vi "GenerateDigitalWaveform.vi"(8 "error in (no error)":errorcluster, 11 "SetupInfo_IN":T1={"ConfigParameters_Analog"={"JAI camera fps"=240.0, "Bi-Lateral Galvo xy scan range (V)"=0.7, "Bi-Lateral Galvo xy scan frequency (Hz)"=500, "AOM Blind percent (%)"=0.1, "AOM start blind percent (%) "=70.0, "ROI threshold"=1.0, "AO Sampling rate"=1000000.0}, "ConfigParameters_Digital"={"Steps per volume"=25.0, "Time per volume (s)"=0.4, "OG start layer"=15.0, "Objective Lin Rising Vel (micron/ms）"=1.0, "Image depth (micron)"=200.0, "OG latency (s)"=10.0, "OG repitation"=3.0, "OG end layer"=17.0, "Shock1 duration (s)"=0.001, "Shock2 duration (s)"=0.001, "Shock3 duration (s)"=0.01, "Shock4 duration (s)"=0.01, "Shock5 duration (s)"=0.1, "Shock duration_New"=[]}, "ConfigParameters_Other1"={"Frontal Galvo xy scan range (V)"=0.14, "Frontal Galvo xy scan frequency (Hz)"=500, "PFI 0 digital clock frequency"=500000.0, "Window size for layer index"=0.5, "sCMOS fps"=95.0}, "ConfigParameters_Others2"={"#Trials baseline"=6, "#Trials test"=6, "Time before acq. (s)"=360.0, "Time before test (s)"=600.0, "#Blocks acquisition"=5, "Inter-trial interval baseline (s)"=60.0, "#Trials per acquition block"=6, "Inter-block interval acquisition (s)"=360.0, "Inter-trial interval acquisition (s)"=20.0, "Flash latency (s)"=10.0, "Flash duration (s)"=3.2, "Response duration (s)"=10.0, "MaxTimeEventDetection (s)"=6, "StimType"=enum."Flash", "#MaxEvents"=6}, "ProcessParametersOut"={"stand Z vol Acquisition time (s)"=0.2631578947368421, "stand Z vol Backward time (s)"=0.13684210526315793, "Objective scan volt"=5.0, "Bi-lateral Galvo Z scan volt"=0.1800000180000018, "Frontal Galvo Z scan volt"=0.14940000509752818, "Objective step length (micron)"=8.0, "OG Z volet Linear Dec time (s)"=0.024, "OG Z vol Stim. steps time (s)"=0.031578947368421054, "OG Z vol Linear Acc time (s)"=0.112, "#Vol. of flash"=8, "#Vol. of shock"=1, "#Vol. bef flash"=25, "#Vol. aft flash"=17, "OG Z vol Linear Dec time (s)"=0.112, "OG Z vol time (s)"=0.39073684210526316, "Stack duration"=[0.001, 0.001, 0.01, 0.01, 0.1], "AOM stand. value size"=400000, "Plane indexing length"=0, "#Vol. blank"=0, "#Vol. blank before acq"=0, "#Vol. blank before test"=0, " #Inter-block interval acquisition (Ed-St Vol)"=0}, "WaveformParameters"={"stand Z vol Acquisition samp info"={"Fs"=1000000.0, "#s"=263158.0}, "stand Z vol Backward samp info"={"Fs"=1000000.0, "#s"=136842.0}, "OG Z vol Linear Acc samp info"={"Fs"=1000000.0, "#s"=112000.0}, "OG Z vol Stim. steps samp info"={"Fs"=1000000.0, "#s"=31579.0}, "OG Z volet Linear Dec samp info"={"Fs"=1000000.0, "#s"=24000.0}, "OG Z vol Linear Dec samp info"={"Fs"=1000000.0, "#s"=112000.0}, "OG Z vol samp info"={"Fs"=1000000.0, "#s"=390737.0}, "stand Z vol backforth samp info"={"Fs"=1000000.0, "#s"=400000.0}}, "AnalogWaveform"={"Bi-lateral Galvo Z stand waveform"={"t0"=timestamp(0 s since 1904-01-01), "dt"=1.0, "Y"=[]}, "Frontal Galvo Z stand waveform"={"t0"=timestamp(0 s since 1904-01-01), "dt"=1.0, "Y"=[]}, "Bi-lateral Galvo XY stand waveform"={"t0"=timestamp(0 s since 1904-01-01), "dt"=1.0, "Y"=[]}, "Frontal Galvo XY stand waveform"={"t0"=timestamp(0 s since 1904-01-01), "dt"=1.0, "Y"=[]}, "sCMOS stand waveform"={"t0"=timestamp(0 s since 1904-01-01), "dt"=1.0, "Y"=[]}, "Detection objective stand waveform"={"t0"=timestamp(0 s since 1904-01-01), "dt"=1.0, "Y"=[]}, "AOM stand waveform"={"t0"=timestamp(0 s since 1904-01-01), "dt"=1.0, "Y"=[]}, "PFI 0 clock stand waveform"={"t0"=timestamp(0 s since 1904-01-01), "dt"=1.0, "Y"=[]}, "Bi-lateral Galvo Z OG waveform"={"t0"=timestamp(0 s since 1904-01-01), "dt"=1.0, "Y"=[]}, "Bi-lateral Galvo XY OG waveform"={"t0"=timestamp(0 s since 1904-01-01), "dt"=1.0, "Y"=[]}, "Frontal Galvo Z OG waveform"={"t0"=timestamp(0 s since 1904-01-01), "dt"=1.0, "Y"=[]}, "Frontal Galvo XY OG waveform"={"t0"=timestamp(0 s since 1904-01-01), "dt"=1.0, "Y"=[]}, "sCMOS OG waveform"={"t0"=timestamp(0 s since 1904-01-01), "dt"=1.0, "Y"=[]}, "Detection objective OG waveform"={"t0"=timestamp(0 s since 1904-01-01), "dt"=1.0, "Y"=[]}, "AOM OG waveform"={"t0"=timestamp(0 s since 1904-01-01), "dt"=1.0, "Y"=[]}, "PFI 0 clock OG wavee"={"t0"=timestamp(0 s since 1904-01-01), "dt"=1.0, "Y"=[]}, "sCMOS blank waveform"={"t0"=timestamp(0 s since 1904-01-01), "dt"=1.0, "Y"=[]}, "All analog OG wave"=[], "All analog stand wave"=[], "All analog blank wave"=[], "BufferWaveform_Analog"=[], "Bi-lateral Galvo Z XY"={"t0"=timestamp(0 s since 1904-01-01), "dt"=1.0, "Y"=[]}, "Frontal Galvo Z XY"={"t0"=timestamp(0 s since 1904-01-01), "dt"=1.0, "Y"=[]}, "sCMOS Trigger XY"={"t0"=timestamp(0 s since 1904-01-01), "dt"=1.0, "Y"=[]}, "Detection objective XY"={"t0"=timestamp(0 s since 1904-01-01), "dt"=1.0, "Y"=[]}, "AOM XY"={"t0"=timestamp(0 s since 1904-01-01), "dt"=1.0, "Y"=[]}, "Analog_XY"=[]}, "DigitalWaveform"={"AllDigitalStandWave"=[], "AllDigialEvokedWave"=[], "AllDigialOGWave"=[], "AllDigitalPairWave_1"=[], "AllDigitalPairWave_2"=[], "AllDigitalPairWave_3"=[], "AllDigitalPairWave_4"=[], "AllDigitalPairWave_5"=[], "Plane Indexing"={"t0"=timestamp(0 s since 1904-01-01), "dt"=0.0, "Y"={"transitions"=[], "data"=[]}, "error"={"status"=FALSE, "code"=37421928, "source"=""}}, "Plane indexing P0.5 OG"={"t0"=timestamp(0 s since 1904-01-01), "dt"=0.0, "Y"={"transitions"=[], "data"=[]}, "error"={"status"=FALSE, "code"=37421928, "source"=""}}, "AllDigitalPairWaves"=[], "BufferWaveform_Digital"=[], "AllDigitalBlankWave"=[], "Digial_XY"=[], "Digital_XY_flash"=[], "Digial_XY DMD"=[]}, "PhysicalResource"={"PhysicalChannels_AI"="", "PhysicalChannels_AO"="", "PhysicalChannels_DO"="", "Task_AnalogOutput"="", "Task_DigitalOutput"="", "Task_AnalogInput"=""}, "ControlsRef"={"Mode_1"=refnum, "EventDetectionMode"=refnum, "Mode_2A"=refnum, "StimulationMode"=refnum, "Mode_2B"=refnum, "ErrorMeg"=refnum}, "test"=""} {"ConfigParameters_Other1"."Frontal Galvo xy scan frequency (Hz)" min=500 max=500; "ConfigParameters_Other1"."Frontal Galvo xy scan range (V)" min=0.0 max=1.5; "ConfigParameters_Analog"."AOM start blind percent (%)" min=10.0 max=90.0; "ConfigParameters_Analog"."AOM Blind percent (%)" min=0.1 max=100.0; "ConfigParameters_Analog"."Bi-Lateral Galvo xy scan frequency (Hz)" min=500 max=500; "ConfigParameters_Analog"."Bi-Lateral Galvo xy scan range (V)" min=0.0 max=1.5}) -> (0 "error out":errorcluster, 3 "SetupInfo_OUT":T1={"ConfigParameters_Analog"={"JAI camera fps"=240.0, "Bi-Lateral Galvo xy scan range (V)"=0.7, "Bi-Lateral Galvo xy scan frequency (Hz)"=500, "AOM Blind percent (%)"=0.1, "AOM start blind percent (%) "=70.0, "ROI threshold"=1.0, "AO Sampling rate"=1000000.0}, "ConfigParameters_Digital"={"Steps per volume"=25.0, "Time per volume (s)"=0.4, "OG start layer"=15.0, "Objective Lin Rising Vel (micron/ms）"=1.0, "Image depth (micron)"=200.0, "OG latency (s)"=10.0, "OG repitation"=3.0, "OG end layer"=17.0, "Shock1 duration (s)"=0.001, "Shock2 duration (s)"=0.001, "Shock3 duration (s)"=0.01, "Shock4 duration (s)"=0.01, "Shock5 duration (s)"=0.1, "Shock duration_New"=[]}, "ConfigParameters_Other1"={"Frontal Galvo xy scan range (V)"=0.14, "Frontal Galvo xy scan frequency (Hz)"=500, "PFI 0 digital clock frequency"=500000.0, "Window size for layer index"=0.5, "sCMOS fps"=95.0}, "ConfigParameters_Others2"={"#Trials baseline"=6, "#Trials test"=6, "Time before acq. (s)"=360.0, "Time before test (s)"=600.0, "#Blocks acquisition"=5, "Inter-trial interval baseline (s)"=60.0, "#Trials per acquition block"=6, "Inter-block interval acquisition (s)"=360.0, "Inter-trial interval acquisition (s)"=20.0, "Flash latency (s)"=10.0, "Flash duration (s)"=3.2, "Response duration (s)"=10.0, "MaxTimeEventDetection (s)"=6, "StimType"=enum."Flash", "#MaxEvents"=6}, "ProcessParametersOut"={"stand Z vol Acquisition time (s)"=0.2631578947368421, "stand Z vol Backward time (s)"=0.13684210526315793, "Objective scan volt"=5.0, "Bi-lateral Galvo Z scan volt"=0.1800000180000018, "Frontal Galvo Z scan volt"=0.14940000509752818, "Objective step length (micron)"=8.0, "OG Z volet Linear Dec time (s)"=0.024, "OG Z vol Stim. steps time (s)"=0.031578947368421054, "OG Z vol Linear Acc time (s)"=0.112, "#Vol. of flash"=8, "#Vol. of shock"=1, "#Vol. bef flash"=25, "#Vol. aft flash"=17, "OG Z vol Linear Dec time (s)"=0.112, "OG Z vol time (s)"=0.39073684210526316, "Stack duration"=[0.001, 0.001, 0.01, 0.01, 0.1], "AOM stand. value size"=400000, "Plane indexing length"=0, "#Vol. blank"=0, "#Vol. blank before acq"=0, "#Vol. blank before test"=0, " #Inter-block interval acquisition (Ed-St Vol)"=0}, "WaveformParameters"={"stand Z vol Acquisition samp info"={"Fs"=1000000.0, "#s"=263158.0}, "stand Z vol Backward samp info"={"Fs"=1000000.0, "#s"=136842.0}, "OG Z vol Linear Acc samp info"={"Fs"=1000000.0, "#s"=112000.0}, "OG Z vol Stim. steps samp info"={"Fs"=1000000.0, "#s"=31579.0}, "OG Z volet Linear Dec samp info"={"Fs"=1000000.0, "#s"=24000.0}, "OG Z vol Linear Dec samp info"={"Fs"=1000000.0, "#s"=112000.0}, "OG Z vol samp info"={"Fs"=1000000.0, "#s"=390737.0}, "stand Z vol backforth samp info"={"Fs"=1000000.0, "#s"=400000.0}}, "AnalogWaveform"={"Bi-lateral Galvo Z stand waveform"={"t0"=timestamp(0 s since 1904-01-01), "dt"=1.0, "Y"=[]}, "Frontal Galvo Z stand waveform"={"t0"=timestamp(0 s since 1904-01-01), "dt"=1.0, "Y"=[]}, "Bi-lateral Galvo XY stand waveform"={"t0"=timestamp(0 s since 1904-01-01), "dt"=1.0, "Y"=[]}, "Frontal Galvo XY stand waveform"={"t0"=timestamp(0 s since 1904-01-01), "dt"=1.0, "Y"=[]}, "sCMOS stand waveform"={"t0"=timestamp(0 s since 1904-01-01), "dt"=1.0, "Y"=[]}, "Detection objective stand waveform"={"t0"=timestamp(0 s since 1904-01-01), "dt"=1.0, "Y"=[]}, "AOM stand waveform"={"t0"=timestamp(0 s since 1904-01-01), "dt"=1.0, "Y"=[]}, "PFI 0 clock stand waveform"={"t0"=timestamp(0 s since 1904-01-01), "dt"=1.0, "Y"=[]}, "Bi-lateral Galvo Z OG waveform"={"t0"=timestamp(0 s since 1904-01-01), "dt"=1.0, "Y"=[]}, "Bi-lateral Galvo XY OG waveform"={"t0"=timestamp(0 s since 1904-01-01), "dt"=1.0, "Y"=[]}, "Frontal Galvo Z OG waveform"={"t0"=timestamp(0 s since 1904-01-01), "dt"=1.0, "Y"=[]}, "Frontal Galvo XY OG waveform"={"t0"=timestamp(0 s since 1904-01-01), "dt"=1.0, "Y"=[]}, "sCMOS OG waveform"={"t0"=timestamp(0 s since 1904-01-01), "dt"=1.0, "Y"=[]}, "Detection objective OG waveform"={"t0"=timestamp(0 s since 1904-01-01), "dt"=1.0, "Y"=[]}, "AOM OG waveform"={"t0"=timestamp(0 s since 1904-01-01), "dt"=1.0, "Y"=[]}, "PFI 0 clock OG wavee"={"t0"=timestamp(0 s since 1904-01-01), "dt"=1.0, "Y"=[]}, "sCMOS blank waveform"={"t0"=timestamp(0 s since 1904-01-01), "dt"=1.0, "Y"=[]}, "All analog OG wave"=[], "All analog stand wave"=[], "All analog blank wave"=[], "BufferWaveform_Analog"=[], "Bi-lateral Galvo Z XY"={"t0"=timestamp(0 s since 1904-01-01), "dt"=1.0, "Y"=[]}, "Frontal Galvo Z XY"={"t0"=timestamp(0 s since 1904-01-01), "dt"=1.0, "Y"=[]}, "sCMOS Trigger XY"={"t0"=timestamp(0 s since 1904-01-01), "dt"=1.0, "Y"=[]}, "Detection objective XY"={"t0"=timestamp(0 s since 1904-01-01), "dt"=1.0, "Y"=[]}, "AOM XY"={"t0"=timestamp(0 s since 1904-01-01), "dt"=1.0, "Y"=[]}, "Analog_XY"=[]}, "DigitalWaveform"={"AllDigitalStandWave"=[], "AllDigialEvokedWave"=[], "AllDigialOGWave"=[], "AllDigitalPairWave_1"=[], "AllDigitalPairWave_2"=[], "AllDigitalPairWave_3"=[], "AllDigitalPairWave_4"=[], "AllDigitalPairWave_5"=[], "Plane Indexing"={"t0"=timestamp(0 s since 1904-01-01), "dt"=0.0, "Y"={"transitions"=[], "data"=[]}, "error"={"status"=FALSE, "code"=37421928, "source"=""}}, "Plane indexing P0.5 OG"={"t0"=timestamp(0 s since 1904-01-01), "dt"=0.0, "Y"={"transitions"=[], "data"=[]}, "error"={"status"=FALSE, "code"=37421928, "source"=""}}, "AllDigitalPairWaves"=[], "BufferWaveform_Digital"=[], "AllDigitalBlankWave"=[], "Digial_XY"=[], "Digital_XY_flash"=[], "Digial_XY DMD"=[]}, "PhysicalResource"={"PhysicalChannels_AI"="", "PhysicalChannels_AO"="", "PhysicalChannels_DO"="", "Task_AnalogOutput"="", "Task_DigitalOutput"="", "Task_AnalogInput"=""}, "ControlsRef"={"Mode_1"=refnum, "EventDetectionMode"=refnum, "Mode_2A"=refnum, "StimulationMode"=refnum, "Mode_2B"=refnum, "ErrorMeg"=refnum}, "test"=""} {"ConfigParameters_Other1"."Frontal Galvo xy scan frequency (Hz)" min=500 max=500; "ConfigParameters_Other1"."Frontal Galvo xy scan range (V)" min=0.0 max=1.5; "ConfigParameters_Analog"."AOM start blind percent (%)" min=10.0 max=90.0; "ConfigParameters_Analog"."AOM Blind percent (%)" min=0.1 max=100.0; "ConfigParameters_Analog"."Bi-Lateral Galvo xy scan frequency (Hz)" min=500 max=500; "ConfigParameters_Analog"."Bi-Lateral Galvo xy scan range (V)" min=0.0 max=1.5})   [LabVIEW 2018]
uses:
  SubVI/SetupInfo.ctl
  SubVI/ConfigParameters_Analog.ctl
  SubVI/ConfigParameters_Digital.ctl
  SubVI/ConfigParameters_Others1.ctl
  SubVI/ConfigParameters_Others2.ctl
  SubVI/ProcessParametersOut.ctl
  SubVI/WaveformParameters.ctl
  SubVI/AnalogWaveform.ctl
  SubVI/DigitalWaveform.ctl
  SubVI/PhysicalResource.ctl
  SubVI/ControlsRef.ctl
panel:
  out "Electric shock US5":bool[](array[boolean])
  out "Electric shock US4":bool[](array[boolean])
  out "Electric shock US3":bool[](array[boolean])
  out "Electric shock US2":bool[](array[boolean])
  out "Electric shock US":bool[](array[boolean])
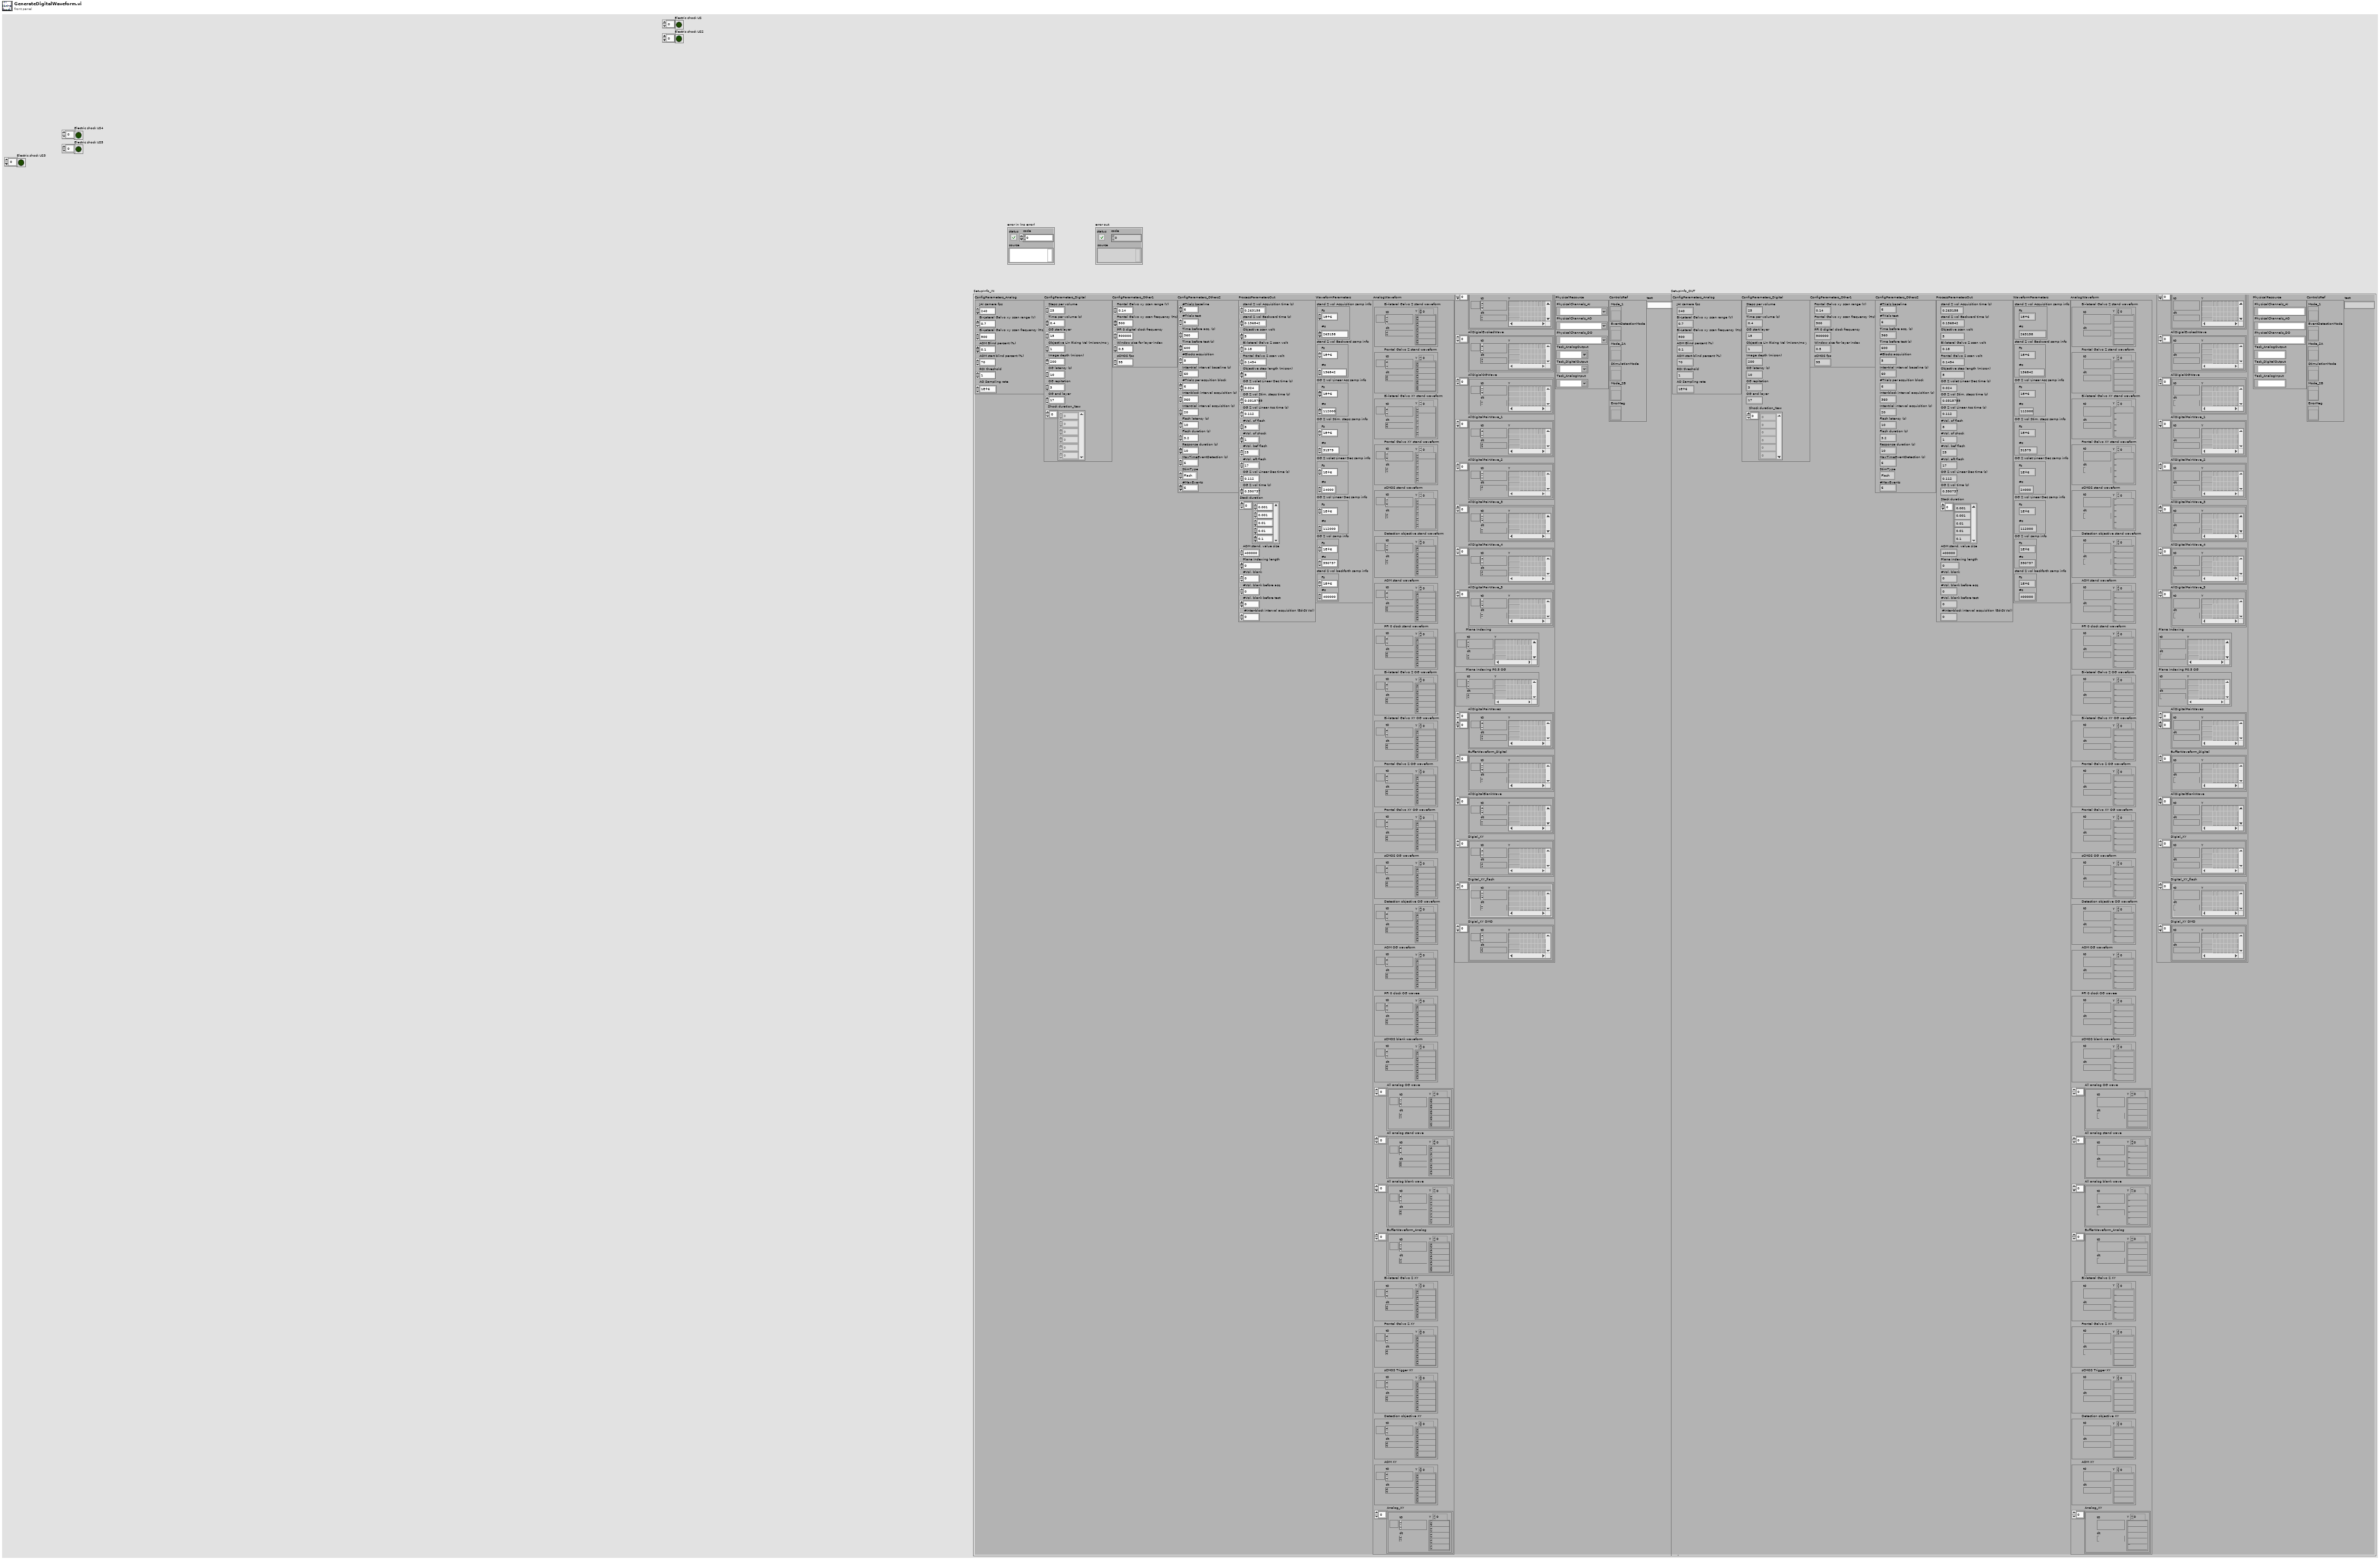
[diagram p1: front panel]
types:
  T1 = typedef "SetupInfo.ctl" = cluster{"ConfigParameters_Analog":T2, "ConfigParameters_Digital":T3, "ConfigParameters_Other1":T4, "ConfigParameters_Others2":T5, "ProcessParametersOut":T6, "WaveformParameters":T7, "AnalogWaveform":T8, "DigitalWaveform":T9, "PhysicalResource":T10, "ControlsRef":T11, "test":string}
  T2 = typedef "ConfigParameters_Analog.ctl" = cluster{"JAI camera fps":dbl, "Bi-Lateral Galvo xy scan range (V)":dbl, "Bi-Lateral Galvo xy scan frequency (Hz)":i16, "AOM Blind percent (%)":dbl, "AOM start blind percent (%) ":dbl, "ROI threshold":dbl, "AO Sampling rate":dbl}
  T3 = typedef "ConfigParameters_Digital.ctl" = cluster{"Steps per volume":dbl, "Time per volume (s)":dbl, "OG start layer":dbl, "Objective Lin Rising Vel (micron/ms）":dbl, "Image depth (micron)":dbl, "OG latency (s)":dbl, "OG repitation":dbl, "OG end layer":dbl, "Shock1 duration (s)":dbl, "Shock2 duration (s)":dbl, "Shock3 duration (s)":dbl, "Shock4 duration (s)":dbl, "Shock5 duration (s)":dbl, "Shock duration_New":dbl[]}
  T4 = typedef "ConfigParameters_Others1.ctl" = cluster{"Frontal Galvo xy scan range (V)":dbl, "Frontal Galvo xy scan frequency (Hz)":i16, "PFI 0 digital clock frequency":dbl, "Window size for layer index":dbl, "sCMOS fps":dbl}
  T5 = typedef "ConfigParameters_Others2.ctl" = cluster{"#Trials baseline":i32, "#Trials test":i32, "Time before acq. (s)":dbl, "Time before test (s)":dbl, "#Blocks acquisition":i32, "Inter-trial interval baseline (s)":dbl, "#Trials per acquition block":i32, "Inter-block interval acquisition (s)":dbl, "Inter-trial interval acquisition (s)":dbl, "Flash latency (s)":dbl, "Flash duration (s)":dbl, "Response duration (s)":dbl, "MaxTimeEventDetection (s)":i32, "StimType":enum16{"Flash", "OG"}, "#MaxEvents":i32}
  T6 = typedef "ProcessParametersOut.ctl" = cluster{"stand Z vol Acquisition time (s)":dbl, "stand Z vol Backward time (s)":dbl, "Objective scan volt":dbl, "Bi-lateral Galvo Z scan volt":dbl, "Frontal Galvo Z scan volt":dbl, "Objective step length (micron)":dbl, "OG Z volet Linear Dec time (s)":dbl, "OG Z vol Stim. steps time (s)":dbl, "OG Z vol Linear Acc time (s)":dbl, "#Vol. of flash":i32, "#Vol. of shock":i32, "#Vol. bef flash":i32, "#Vol. aft flash":i32, "OG Z vol Linear Dec time (s)":dbl, "OG Z vol time (s)":dbl, "Stack duration":dbl[], "AOM stand. value size":i32, "Plane indexing length":i32, "#Vol. blank":i32, "#Vol. blank before acq":i32, "#Vol. blank before test":i32, " #Inter-block interval acquisition (Ed-St Vol)":i32}
  T7 = typedef "WaveformParameters.ctl" = cluster{"stand Z vol Acquisition samp info":cluster{"Fs":dbl, "#s":dbl}, "stand Z vol Backward samp info":cluster{"Fs":dbl, "#s":dbl}, "OG Z vol Linear Acc samp info":cluster{"Fs":dbl, "#s":dbl}, "OG Z vol Stim. steps samp info":cluster{"Fs":dbl, "#s":dbl}, "OG Z volet Linear Dec samp info":cluster{"Fs":dbl, "#s":dbl}, "OG Z vol Linear Dec samp info":cluster{"Fs":dbl, "#s":dbl}, "OG Z vol samp info":cluster{"Fs":dbl, "#s":dbl}, "stand Z vol backforth samp info":cluster{"Fs":dbl, "#s":dbl}}
  T8 = typedef "AnalogWaveform.ctl" = cluster{"Bi-lateral Galvo Z stand waveform":waveform(dbl), "Frontal Galvo Z stand waveform":waveform(dbl), "Bi-lateral Galvo XY stand waveform":waveform(dbl), "Frontal Galvo XY stand waveform":waveform(dbl), "sCMOS stand waveform":waveform(dbl), "Detection objective stand waveform":waveform(dbl), "AOM stand waveform":waveform(dbl), "PFI 0 clock stand waveform":waveform(dbl), "Bi-lateral Galvo Z OG waveform":waveform(dbl), "Bi-lateral Galvo XY OG waveform":waveform(dbl), "Frontal Galvo Z OG waveform":waveform(dbl), "Frontal Galvo XY OG waveform":waveform(dbl), "sCMOS OG waveform":waveform(dbl), "Detection objective OG waveform":waveform(dbl), "AOM OG waveform":waveform(dbl), "PFI 0 clock OG wavee":waveform(dbl), "sCMOS blank waveform":waveform(dbl), "All analog OG wave":waveform(dbl)[], "All analog stand wave":waveform(dbl)[], "All analog blank wave":waveform(dbl)[], "BufferWaveform_Analog":waveform(dbl)[], "Bi-lateral Galvo Z XY":waveform(dbl), "Frontal Galvo Z XY":waveform(dbl), "sCMOS Trigger XY":waveform(dbl), "Detection objective XY":waveform(dbl), "AOM XY":waveform(dbl), "Analog_XY":waveform(dbl)[]}
  T9 = typedef "DigitalWaveform.ctl" = cluster{"AllDigitalStandWave":digitalwaveform[], "AllDigialEvokedWave":digitalwaveform[], "AllDigialOGWave":digitalwaveform[], "AllDigitalPairWave_1":digitalwaveform[], "AllDigitalPairWave_2":digitalwaveform[], "AllDigitalPairWave_3":digitalwaveform[], "AllDigitalPairWave_4":digitalwaveform[], "AllDigitalPairWave_5":digitalwaveform[], "Plane Indexing":digitalwaveform, "Plane indexing P0.5 OG":digitalwaveform, "AllDigitalPairWaves":digitalwaveform[][], "BufferWaveform_Digital":digitalwaveform[], "AllDigitalBlankWave":digitalwaveform[], "Digial_XY":digitalwaveform[], "Digital_XY_flash":digitalwaveform[], "Digial_XY DMD":digitalwaveform[]}
  T10 = typedef "PhysicalResource.ctl" = cluster{"PhysicalChannels_AI":tag, "PhysicalChannels_AO":tag, "PhysicalChannels_DO":tag, "Task_AnalogOutput":refnum<k21>, "Task_DigitalOutput":refnum<k21>, "Task_AnalogInput":refnum<k21>}
  T11 = typedef "ControlsRef.ctl" = cluster{"Mode_1":refnum<vi>, "EventDetectionMode":refnum<vi>, "Mode_2A":refnum<vi>, "StimulationMode":refnum<vi>, "Mode_2B":refnum<vi>, "ErrorMeg":refnum<vi>}
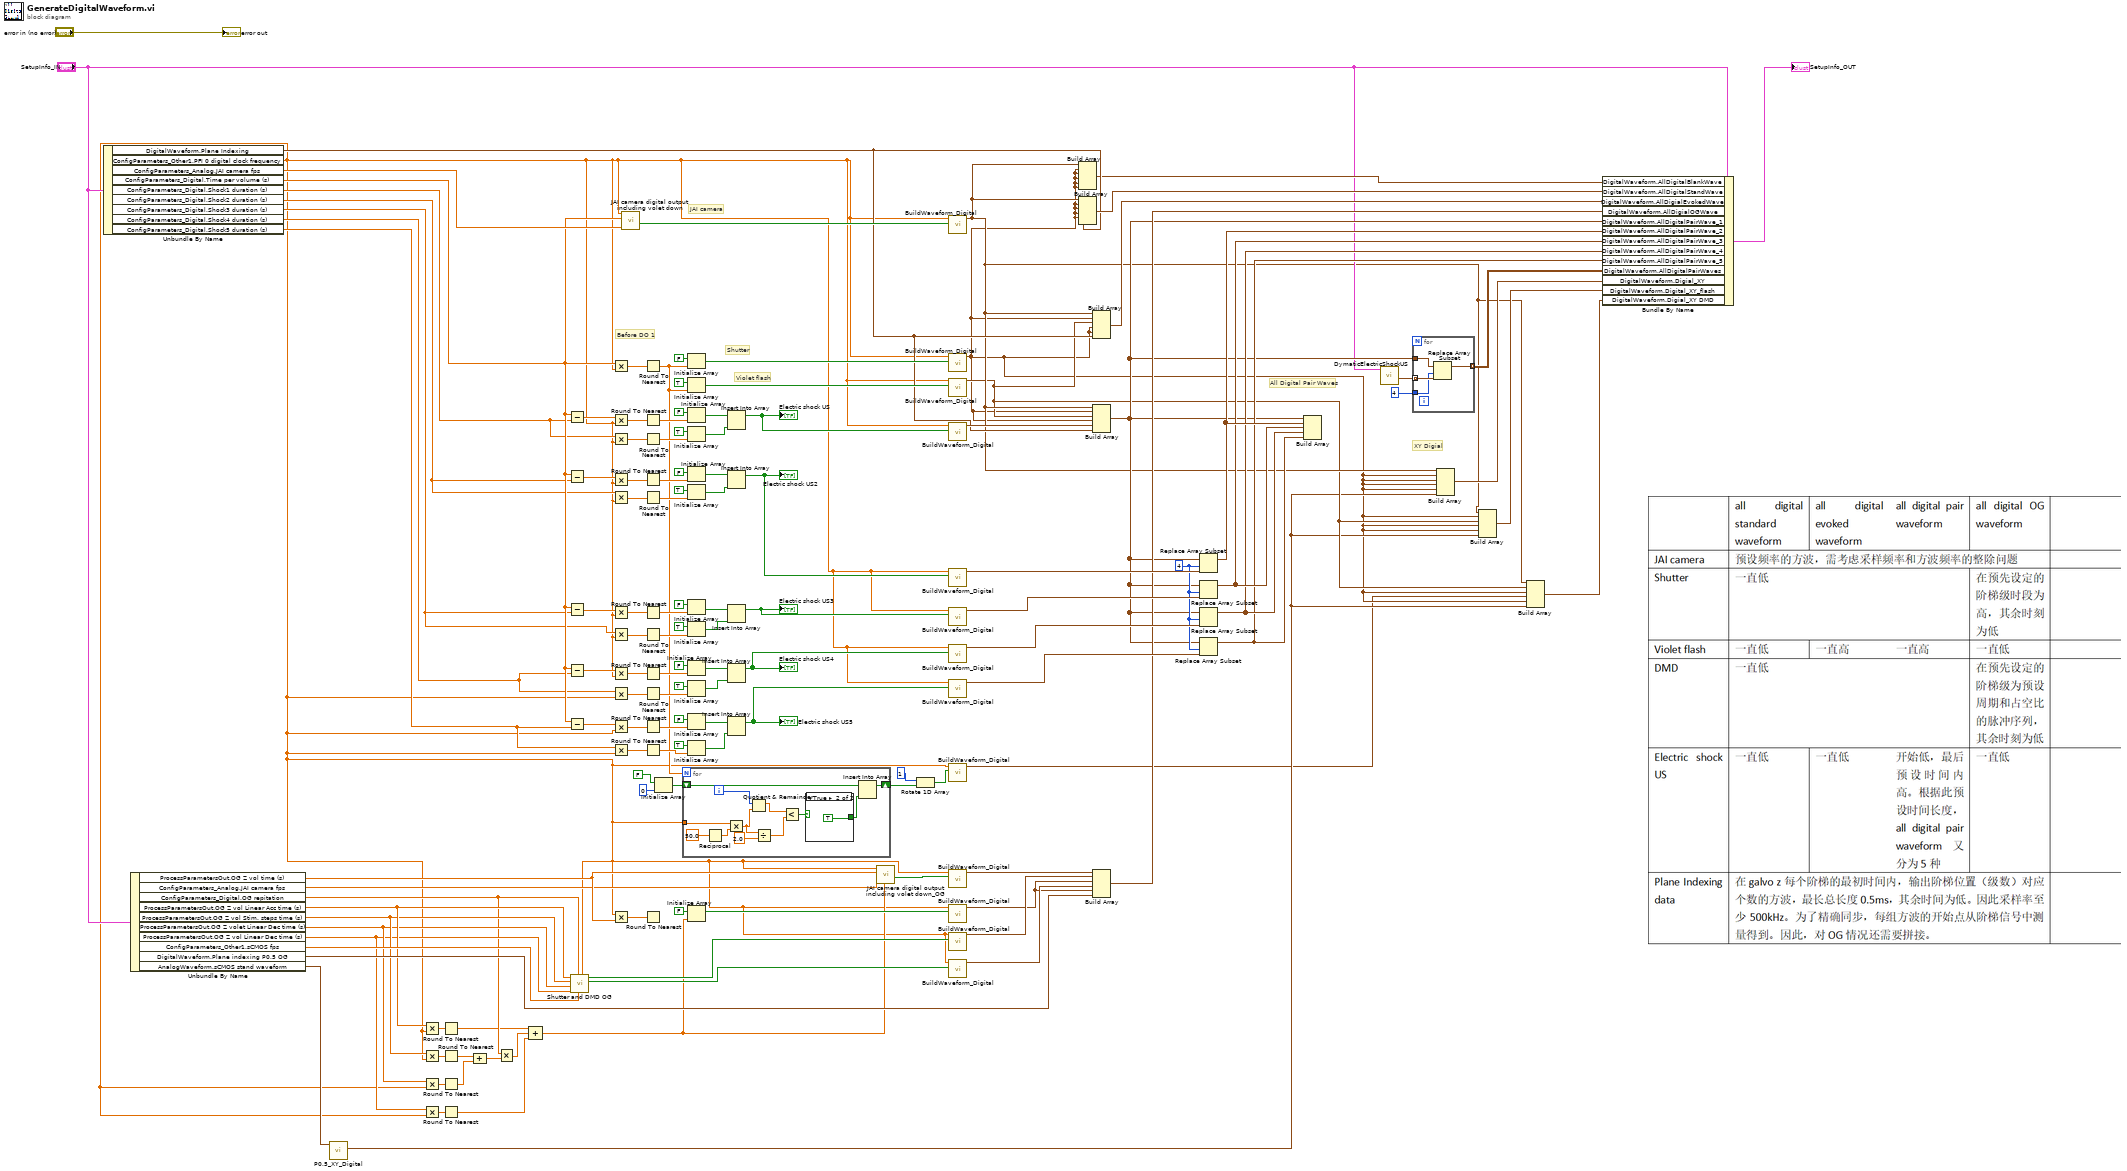
[diagram p0: block diagram]
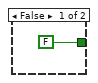
[diagram p2: hidden frame]
diagram:
  w51 = 4 ("index")
  # "XY Digial"
  # "All Digital Pair Waves"
  # "Violet flash"
  # "Shutter"
  # "JAI camera"
  # "Before DO 1"
  n1 = Unbundle By Name("SetupInfo_IN") -> ("DigitalWaveform.Plane Indexing"=w48:digitalwaveform, "ConfigParameters_Other1.PFI 0 digital clock frequency"=w8:dbl, "ConfigParameters_Analog.JAI camera fps"=w84:dbl, "ConfigParameters_Digital.Time per volume (s)"=w83:dbl, "ConfigParameters_Digital.Shock1 duration (s)"=w82:dbl, "ConfigParameters_Digital.Shock2 duration (s)"=w81:dbl, "ConfigParameters_Digital.Shock3 duration (s)"=w80:dbl, "ConfigParameters_Digital.Shock4 duration (s)"=w79:dbl, "ConfigParameters_Digital.Shock5 duration (s)"=w78:dbl)
  n2 = Unbundle By Name("SetupInfo_IN") -> ("ProcessParametersOut.OG Z vol time (s)"=w26:dbl, "ConfigParameters_Analog.JAI camera fps"=w25:dbl, "ConfigParameters_Digital.OG repitation"=w30:dbl, "ProcessParametersOut.OG Z vol Linear Acc time (s)"=w40:dbl, "ProcessParametersOut.OG Z vol Stim. steps time (s)"=w36:dbl, "ProcessParametersOut.OG Z volet Linear Dec time (s)"=w35:dbl, "ProcessParametersOut.OG Z vol Linear Dec time (s)"=w34:dbl, "ConfigParameters_Other1.sCMOS fps"=w62:dbl, "DigitalWaveform.Plane indexing P0.5 OG"=w57:digitalwaveform, "AnalogWaveform.sCMOS stand waveform"=w16:waveform(dbl))
  n3 = call "P0.5_XY_Digital.vi"("In"=w16) -> ("P0.5_Digital_XY"=w12:digitalwaveform)  [unwired: 9 in, 1 out]
  n4 = Multiply(x=w40, y=w8) -> (x*y=w41:dbl)
  n5 = Multiply(x=w36, y=w8) -> (x*y=w39:dbl)
  n6 = Multiply(x=w35, y=w8) -> (x*y=w38:dbl)
  n7 = Multiply(x=w34, y=w8) -> (x*y=w37:dbl)
  n8 = Round To Nearest(number=w41) -> (nearest integer value=w29:dbl)
  n9 = Round To Nearest(number=w39) -> (nearest integer value=w33:dbl)
  n10 = Round To Nearest(number=w38) -> (nearest integer value=w32:dbl)
  n11 = Round To Nearest(number=w37) -> (nearest integer value=w27:dbl)
  n12 = Compound Arithmetic op=ADD(w33, w32) -> (w31:dbl)
  n13 = Multiply(x=w30, y=w31) -> (x*y=w28:dbl)
  n14 = Compound Arithmetic op=ADD(w29, w28, w27) -> (w24:dbl)
  n15 = Subtract(x=w83, y=w82) -> (x-y=w127:dbl)
  n16 = Subtract(x=w83, y=w81) -> (x-y=w126:dbl)
  n17 = Subtract(x=w83, y=w80) -> (x-y=w105:dbl)
  n18 = Subtract(x=w83, y=w79) -> (x-y=w104:dbl)
  n19 = Subtract(x=w83, y=w78) -> (x-y=w103:dbl)
  n20 = call "Shutter and DMD OG.vi"("PFI 0 digital clock frequency"=w8, "sCMOS fps"=w62, "OG repitation"=w30, "Objective 线性减速 时间（s）"=w34, "Objective volet 线性减速 时间（s）"=w35, "Objective 刺激steps 时间（s）"=w36, "Objective 线性加速 时间（s）"=w40) -> ("DMD OG digital output"=w42:bool[], "Shutter OG digital output"=w61:bool[])  [unwired: 2 in]
  n21 = Multiply(x=w83, y=w8) -> (x*y=w132:dbl)
  n22 = Multiply(x=w127, y=w8) -> (x*y=w131:dbl)
  n23 = Multiply(x=w82, y=w8) -> (x*y=w130:dbl)
  n24 = Multiply(x=w126, y=w8) -> (x*y=w129:dbl)
  n25 = Multiply(x=w81, y=w8) -> (x*y=w128:dbl)
  n26 = Multiply(x=w105, y=w8) -> (x*y=w111:dbl)
  n27 = Multiply(x=w80, y=w8) -> (x*y=w110:dbl)
  n28 = Multiply(x=w104, y=w8) -> (x*y=w109:dbl)
  n29 = Multiply(x=w79, y=w8) -> (x*y=w108:dbl)
  n30 = Multiply(x=w103, y=w8) -> (x*y=w107:dbl)
  n31 = Multiply(x=w78, y=w8) -> (x*y=w106:dbl)
  n32 = Multiply(x=w8, y=w26) -> (x*y=w64:dbl)
  n33 = call "JAI camera digital output including volet down.vi"("JAI camera fps"=w84, "OG volAcquisitionTime"=w83, "PFI 0 digital clock frequency"=w8) -> ("JAI camera digital output"=w73:bool[])  [unwired: 8 in]
  n34 = Round To Nearest(number=w132) -> (nearest integer value=w9:dbl)
  n35 = Round To Nearest(number=w131) -> (nearest integer value=w125:dbl)
  n36 = Round To Nearest(number=w130) -> (nearest integer value=w124:dbl)
  n37 = Round To Nearest(number=w129) -> (nearest integer value=w123:dbl)
  n38 = Round To Nearest(number=w128) -> (nearest integer value=w122:dbl)
  n39 = Round To Nearest(number=w111) -> (nearest integer value=w102:dbl)
  n40 = Round To Nearest(number=w110) -> (nearest integer value=w101:dbl)
  n41 = Round To Nearest(number=w109) -> (nearest integer value=w100:dbl)
  n42 = Round To Nearest(number=w108) -> (nearest integer value=w99:dbl)
  n43 = Round To Nearest(number=w107) -> (nearest integer value=w98:dbl)
  n44 = Round To Nearest(number=w106) -> (nearest integer value=w97:dbl)
  n45 = Round To Nearest(number=w64) -> ()  [unwired: 1 out]
  n46 = Initialize Array(FALSE, 0 ("dimension size")) -> (w5:bool[])
  n47 = for {
    N: w9 -> [_]
    tunnel: w8 -> [w144]
    shift-right: [w134] -> w4
    shift-left: w5 -> [w135]
    i -> [w142]
    n48 = Reciprocal(x=50.0) -> (1/x=w143:dbl)
    n49 = Multiply(x=w144, y=w143) -> (x*y=w140:dbl)
    n50 = Quotient & Remainder(x=w142, y=w140) -> (x-y*floor(x/y)=w141:dbl)  [unwired: 1 out]
    n51 = Divide(x=w140, y=2.0) -> (x/y=w138:dbl)
    n52 = Less?(x=w141, y=w138) -> (x < y?=w137:bool)
    n53 = case shown="True" w137 {
      tunnel: [FALSE TRUE] -> w136
      frame False {
      }
      frame True {
      }
    }
    n54 = Insert Into Array(array=w135, new element=w136) -> (w134:bool[])  [unwired: 1 in]
  }
  n55 = Initialize Array(FALSE, w9) -> (w72:bool[])
  n56 = Initialize Array(TRUE, w9) -> (w71:bool[])
  n57 = Initialize Array(FALSE, w125) -> (w114:bool[])
  n58 = Initialize Array(TRUE, w124) -> (w115:bool[])
  n59 = Initialize Array(FALSE, w123) -> (w113:bool[])
  n60 = Initialize Array(TRUE, w122) -> (w112:bool[])
  n61 = Initialize Array(FALSE, w102) -> (w86:bool[])
  n62 = Initialize Array(TRUE, w101) -> (w85:bool[])
  n63 = Initialize Array(FALSE, w100) -> (w88:bool[])
  n64 = Initialize Array(TRUE, w99) -> (w87:bool[])
  n65 = Initialize Array(FALSE, w98) -> (w90:bool[])
  n66 = Initialize Array(TRUE, w97) -> (w89:bool[])
  n67 = Initialize Array(FALSE, w24) -> (w63:bool[])
  n68 = Insert Into Array(array=w114, new element=w115) -> (w70:bool[])  [unwired: 1 in]
  "Electric shock US" <- w70
  n69 = Insert Into Array(array=w113, new element=w112) -> (w69:bool[])  [unwired: 1 in]
  "Electric shock US2" <- w69
  n70 = Insert Into Array(array=w86, new element=w85) -> (w74:bool[])  [unwired: 1 in]
  "Electric shock US3" <- w74
  n71 = Insert Into Array(array=w88, new element=w87) -> (w68:bool[])  [unwired: 1 in]
  "Electric shock US4" <- w68
  n72 = Insert Into Array(array=w90, new element=w89) -> (w67:bool[])  [unwired: 1 in]
  "Electric shock US5" <- w67
  n73 = call "JAI camera digital output including volet down_OG.vi"("AllSize"=w24, "JAI camera fps"=w25, "OG volAcquisitionTime"=w26, "PFI 0 digital clock frequency"=w8) -> ("JAI camera digital output"=w23:bool[])  [unwired: 7 in]
  n74 = Rotate 1D Array(1:w4, 2:1 ("n")) -> (0:w3:bool[])
  n75 = call "BuildWaveform_Digital.vi"("DigitalData"=w73, "SampleRate"=w8) -> ("DigitalWaveformOut"=w14:digitalwaveform)  [unwired: 9 in]
  n76 = call "BuildWaveform_Digital.vi"("DigitalData"=w72, "SampleRate"=w8) -> ("DigitalWaveformOut"=w11:digitalwaveform)  [unwired: 9 in]
  n77 = call "BuildWaveform_Digital.vi"("DigitalData"=w71, "SampleRate"=w8) -> ("DigitalWaveformOut"=w13:digitalwaveform)  [unwired: 9 in]
  n78 = call "BuildWaveform_Digital.vi"("DigitalData"=w70, "SampleRate"=w8) -> ("DigitalWaveformOut"=w49:digitalwaveform)  [unwired: 9 in]
  n79 = call "BuildWaveform_Digital.vi"("DigitalData"=w69, "SampleRate"=w8) -> ("DigitalWaveformOut"=w55:digitalwaveform)  [unwired: 9 in]
  n80 = call "BuildWaveform_Digital.vi"("DigitalData"=w74, "SampleRate"=w8) -> ("DigitalWaveformOut"=w54:digitalwaveform)  [unwired: 9 in]
  n81 = call "BuildWaveform_Digital.vi"("DigitalData"=w68, "SampleRate"=w8) -> ("DigitalWaveformOut"=w53:digitalwaveform)  [unwired: 9 in]
  n82 = call "BuildWaveform_Digital.vi"("DigitalData"=w67, "SampleRate"=w8) -> ("DigitalWaveformOut"=w52:digitalwaveform)  [unwired: 9 in]
  n83 = call "BuildWaveform_Digital.vi"("DigitalData"=w3, "SampleRate"=w8) -> ("DigitalWaveformOut"=w10:digitalwaveform)  [unwired: 9 in]
  n84 = call "BuildWaveform_Digital.vi"("DigitalData"=w23, "SampleRate"=w8) -> ("DigitalWaveformOut"=w66:digitalwaveform)  [unwired: 9 in]
  n85 = call "BuildWaveform_Digital.vi"("DigitalData"=w63, "SampleRate"=w8) -> ("DigitalWaveformOut"=w58:digitalwaveform)  [unwired: 9 in]
  n86 = call "BuildWaveform_Digital.vi"("DigitalData"=w61, "SampleRate"=w8) -> ("DigitalWaveformOut"=w60:digitalwaveform)  [unwired: 9 in]
  n87 = call "BuildWaveform_Digital.vi"("DigitalData"=w42, "SampleRate"=w8) -> ("DigitalWaveformOut"=w59:digitalwaveform)  [unwired: 9 in]
  n88 = Build Array(w14, w11, w11, w11, w11, w11) -> (w43:digitalwaveform[])
  n89 = Build Array(w14, w11, w11, w11, w11, w48) -> (w76:digitalwaveform[])
  n90 = Build Array(w14, w11, w13, w11, w11, w48) -> (w75:digitalwaveform[])
  n91 = Build Array(w14, w11, w13, w11, w49, w48) -> (w21:digitalwaveform[])
  n92 = Build Array(w66, w60, w58, w59, w58, w57) -> (w50:digitalwaveform[])
  n93 = Replace Array Subset(array=w21, new element=w55, index=w51) -> (w47:digitalwaveform[])
  n94 = Replace Array Subset(array=w21, new element=w54, index=w51) -> (w46:digitalwaveform[])
  n95 = Replace Array Subset(array=w21, new element=w53, index=w51) -> (w45:digitalwaveform[])
  n96 = Replace Array Subset(array=w21, new element=w52, index=w51) -> (w44:digitalwaveform[])
  n97 = Build Array(w21, w47, w46, w45, w44) -> ()  [unwired: 1 out]
  n98 = call "DymaticElectricShockUS.vi"("SetupInfo_IN"="SetupInfo_IN") -> ("ElectricShockUS_Out"=w22:digitalwaveform[])  [unwired: 8 in, 2 out]
  n99 = for {
    tunnel: w22 -> [w150] mode=indexing
    tunnel: w21 -> [w149]
    tunnel: 4 ("index") -> [w148]
    tunnel: [w147] -> w19 mode=indexing
    n100 = Replace Array Subset(array=w149, new element=w150, index=w148) -> (w147:digitalwaveform[])
  }
  n101 = Build Array(w14, w11, w11, w11, w11, w12) -> (w17:digitalwaveform[])
  n102 = Build Array(w14, w11, w13, w11, w11, w12) -> (w15:digitalwaveform[])
  n103 = Build Array(w14, w13, w11, w10, w11, w12) -> (w1:digitalwaveform[])
  n104 = Bundle By Name(cluster="SetupInfo_IN", "DigitalWaveform.AllDigitalBlankWave"=w43, "DigitalWaveform.AllDigitalStandWave"=w76, "DigitalWaveform.AllDigialEvokedWave"=w75, "DigitalWaveform.AllDigialOGWave"=w50, "DigitalWaveform.AllDigitalPairWave_1"=w21, "DigitalWaveform.AllDigitalPairWave_2"=w47, "DigitalWaveform.AllDigitalPairWave_3"=w46, "DigitalWaveform.AllDigitalPairWave_4"=w45, "DigitalWaveform.AllDigitalPairWave_5"=w44, "DigitalWaveform.AllDigitalPairWaves"=w19, "DigitalWaveform.Digial_XY"=w17, "DigitalWaveform.Digital_XY_flash"=w15, "DigitalWaveform.Digial_XY DMD"=w1) -> (→"SetupInfo_OUT":T1)
  "error out" <- "error in (no error)"
